vi "appendFilenameIndex.vi"(8 "newFile? (no:F)":bool, 11 "dup path":path) -> (3 "appended path":path)   [LabVIEW 2021]
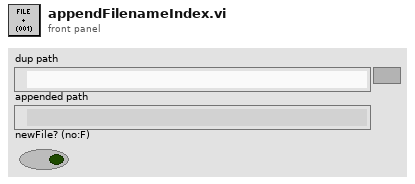
[diagram p1: front panel]
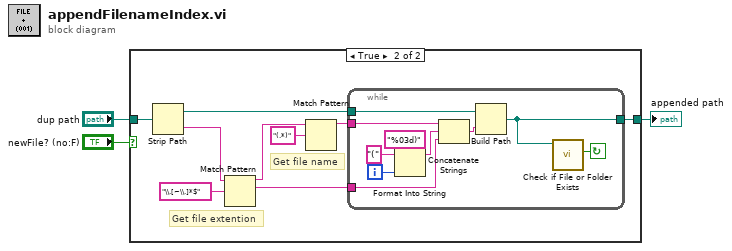
[diagram p0: block diagram]
diagram:
  n1 = case shown="True" "newFile? (no:F)" {
    tunnel: [w4 w13] -> w2
    tunnel: "dup path" -> [w4 w11]
    frame False {
    }
    frame True {
      # "Get file name"
      # "Get file extention"
      n2 = Strip Path(path=w11) -> (stripped path=w12:path, name=w8:string)
      n3 = Match Pattern(string=w8, regular expression="\\.[~\\.]*$") -> (before substring=w7:string, match substring=w9:string)  [unwired: 3 out]
      n4 = Match Pattern(string=w7, regular expression="(.*)") -> (before substring=w6:string)  [unwired: 4 out]
      n5 = while {
        tunnel: [w15] -> w13
        tunnel: w12 -> [w22]
        tunnel: w6 -> [w21]
        tunnel: w9 -> [w16]
        i -> [w14]
        stop <- w23 continue-if-true
        n6 = Format Into String(format string="%03d)", initial string="(", w14) -> (resulting string=w20:string)  [unwired: 1 in, 1 out]
        n7 = Concatenate Strings(w21, w20, w16) -> (w17:string)
        n8 = Build Path(base path=w22, name or relative path=w17) -> (appended path=w15:path)
        n9 = call <vilib>:"Check if File or Folder Exists.vi"("path"=w15) -> ("file or folder exists?"=w23:bool)  [unwired: 8 in, 2 out]
      }
    }
  }
  "appended path" <- w2
